vi "SIM Ros W Factor.vi"(10 "step size":dbl, 11 "Ros data":T1) -> (0 "error":bool, 3 "Ros data out":T1)   [LabVIEW 2017]
uses:
  SIM Rosenbrock data.ctl
  SIM Factored Matrix.ctl
  SIM Ros stages.ctl
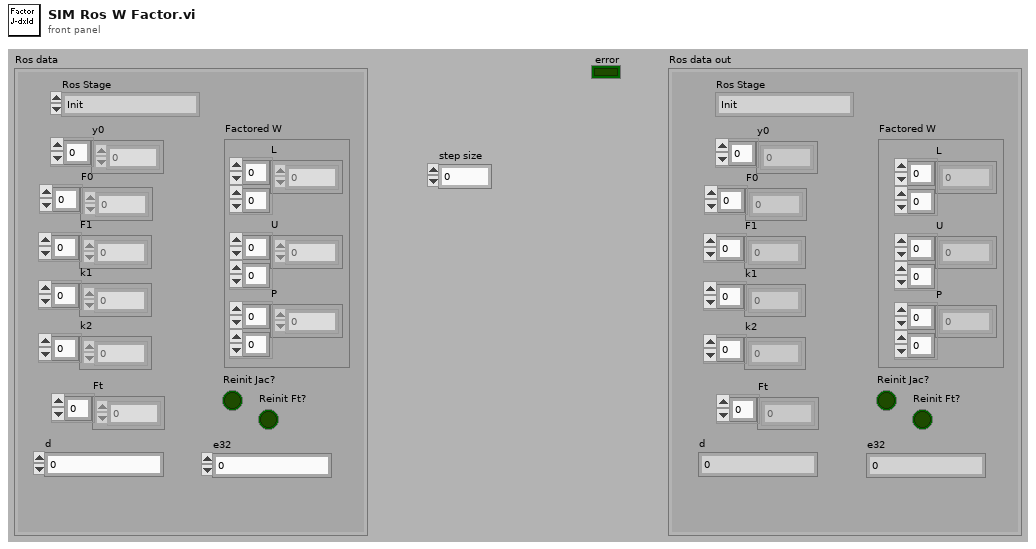
[diagram p1: front panel]
types:
  T1 = typedef "SIM Rosenbrock data.ctl" = cluster{"y0":dbl[], "F0":dbl[], "F1":dbl[], "k1":dbl[], "k2":dbl[], "Factored W":T2, "Ros Stage":T3, "Ft":dbl[], "Reinit Jac?":bool, "Reinit Ft?":bool, "d":dbl, "e32":dbl}
  T2 = typedef "SIM Factored Matrix.ctl" = cluster{"L":dbl[][], "U":dbl[][], "P":i32[][]}
  T3 = typedef "SIM Ros stages.ctl" = enum16{"Init", "Compute Jacobian", "Compute Ft", "Compute k1", "Compute k2", "Eval Error", "Choose StepSize", "Reset Integrator"}
  T4 = typedef "NI_Matrix.lvlib/RealMatrix.ctl" = dbl[][]
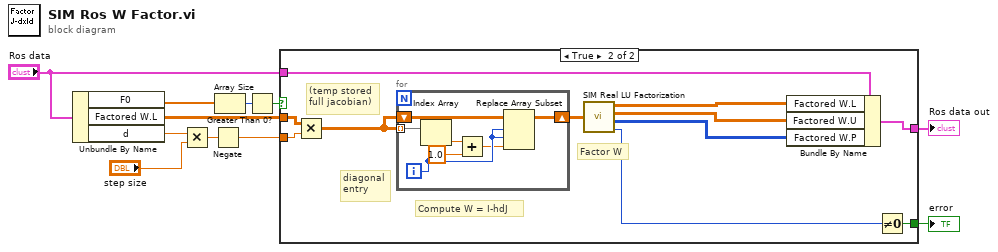
[diagram p0: block diagram]
diagram:
  n1 = Unbundle By Name("Ros data") -> ("F0"=w8:dbl[], "Factored W.L"=w2:dbl[][], "d"=w5:dbl)
  n2 = Multiply(x=w5, y="step size") -> (x*y=w3:dbl)
  n3 = Negate(x=w3) -> (-x=w1:dbl)
  n4 = Array Size(array=w8) -> (size(s)=w7:i32)
  n5 = Greater Than 0?(x=w7) -> (x > 0?=w6:bool)
  n6 = case shown="True" w6 {
    tunnel: [w12 w23] -> w11
    tunnel: [_ w22] -> w10
    tunnel: "Ros data" -> [w12 w21]
    tunnel: w2 -> [_ w19]
    tunnel: w1 -> [_ w20]
    frame False {
    }
    frame True {
      # "Factor W"
      # "Compute W = I-hdJ"
      # "diagonal\nentry"
      # "(temp stored\nfull jacobian)"
      n7 = Multiply(x=w19, y=w20) -> (x*y=w18:dbl[][])
      n8 = for {
        shift-right: [w27] -> w17
        shift-left: w18 -> [w28]
        tunnel: w18 -> [w30] mode=indexing
        i -> [w26]
        n9 = Index Array(array=w30, index=w26) -> (element=w29:dbl)
        n10 = Add(x=w29, y=1.0) -> (x+y=w25:dbl)
        n11 = Replace Array Subset(array=w28, new element=w25, index (row)=w26, index (col)=w26) -> (w27:dbl[][])
      }
      n12 = call "SIM Real LU Factorization.vi"("A"=w17) -> ("L"=w16:T4, "U"=w15:T4, "P"=w14:i32[][], "error"=w13:i32)
      n13 = Bundle By Name(cluster=w21, "Factored W.L"=w16, "Factored W.U"=w15, "Factored W.P"=w14) -> (w23:T1)
      n14 = Not Equal To 0?(x=w13) -> (x != 0?=w22:bool)
    }
  }
  "error" <- w10
  "Ros data out" <- w11
